vi "XLP80_FGlob_DI.vi"(5 "Function (Recall One)":T1=enum."Recall one", 7 "PXI DI Item":i32, 8 "err in":errorcluster caption="error", 10 "DI Values IN":bool[](array[boolean]), 11 "DI Value IN":bool) -> (0 "err out":errorcluster caption="error", 2 "DI Values OUT":bool[](array[boolean]), 3 "DI Value OUT":bool)   [LabVIEW 2021]
uses:
  1886_FGlob_TDefs_Enum_FGlobItems.ctl
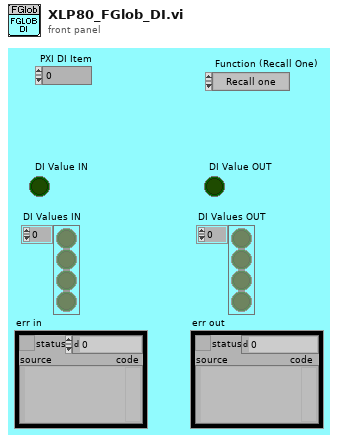
[diagram p1: front panel]
types:
  T1 = typedef "1886_FGlob_TDefs_Enum_FGlobItems.ctl" = enum16{"Put one", "Put all", "Recall one", "Recall all"}
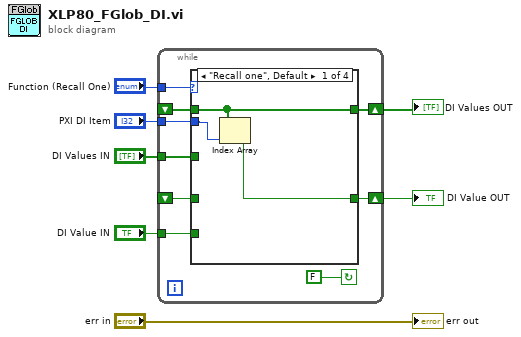
[diagram p0: block diagram]
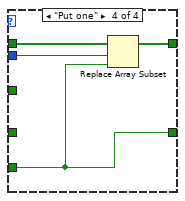
[diagram p4: hidden frame]
diagram:
  n1 = while {
    shift-right: [w14] -> w5
    shift-left: _ -> [w13]
    tunnel: "Function (Recall One)" -> [w15]
    tunnel: "PXI DI Item" -> [w11]
    tunnel: "DI Values IN" -> [w10]
    shift-right: [w12] -> w4
    shift-left: _ -> [w9]
    tunnel: "DI Value IN" -> [w8]
    stop <- FALSE continue-if-true
    n2 = case shown="\"Recall one\", Default" w15 {
      tunnel: [w19 w21 w23 w26] -> w14
      tunnel: w13 -> [w19 w21 _ w27]
      tunnel: w11 -> [w18 _ _ w25]
      tunnel: [w17 w20 w22 w24] -> w12
      tunnel: w10 -> [_ _ w23 _]
      tunnel: w9 -> [_ w20 w22 _]
      tunnel: w8 -> [_ _ _ w24]
      frame "Recall one", Default {
        n3 = Index Array(array=w19, index=w18) -> (element=w17:bool)
      }
      frame "Recall all" {
      }
      frame "Put all" {
      }
      frame "Put one" {
        n4 = Replace Array Subset(array=w27, new element=w24, index=w25) -> (w26:bool[])
      }
    }
  }
  "DI Values OUT" <- w5
  "DI Value OUT" <- w4
  "err out" <- "err in"
